vi "IEEE754-V1.1.vi"(3 "error in (no error)":errorcluster caption="错误输入（无错误）", 5 "数字":i32 format="%.0x") -> (0 "error out":errorcluster caption="错误输出", 2 "输出浮点型":dbl)   [LabVIEW 2015]
panel:
  out "HexFormat":i32=1130102784 format="%x"
  # "IEEE754 2个16位整型转换为浮点型"
  # "1、程序将两个16位整型转换为一个32为的浮点型数据，转换原则按照IEEE754标准进行；\n2、高16、低16位和合并后的Hex格式数据都是16进制显示；\n3、输出浮点型是转换后的数据。"
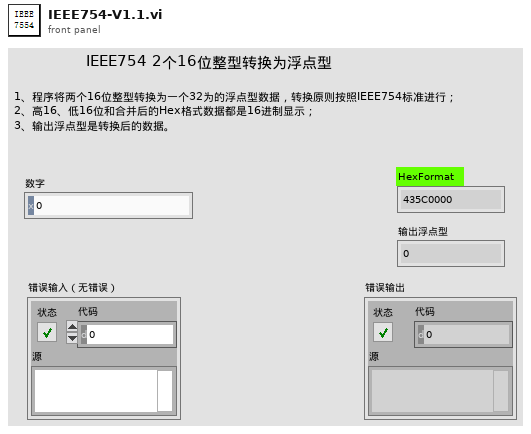
[diagram p1: front panel]
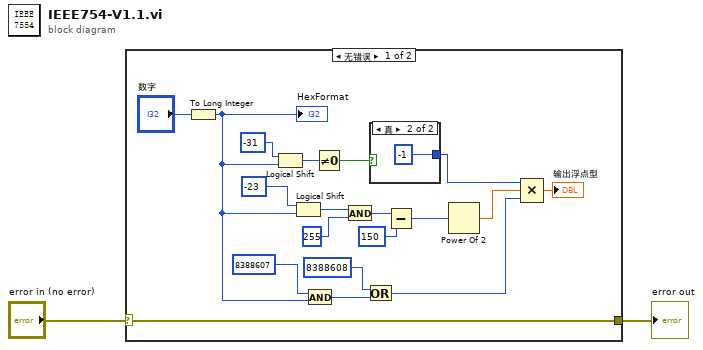
[diagram p0: block diagram]
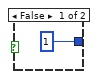
[diagram p2: hidden frame]
diagram:
  n1 = case shown="无错误" "error in (no error)" {
    selector: "error in (no error)" -> [w3 w24]
    tunnel: [w3 w24] -> w1
    frame No Error {
      n2 = To Long Integer(number="数字") -> (32bit integer=w5:i32)
      "HexFormat" <- w5
      n3 = Logical Shift(y=-31, x=w5) -> (x << y=w20:i32)
      n4 = Logical Shift(y=-23, x=w5) -> (x << y=w17:i32)
      n5 = And(x=8388607, y=w5) -> (x .and. y?=w12:i32)
      n6 = Not Equal To 0?(x=w20) -> (x != 0?=w19:bool)
      n7 = And(x=w17, y=255) -> (x .and. y?=w15:i32)
      n8 = Or(x=8388608, y=w12) -> (x .or. y?=w9:i32)
      n9 = case shown="真" w19 {
        tunnel: [1 -1] -> w10
        frame False {
        }
        frame True {
        }
      }
      n10 = Subtract(x=w15, y=150) -> (x-y=w7:i32)
      n11 = Power Of 2(x=w7) -> (2^x=w6:dbl)
      n12 = Compound Arithmetic op=MULTIPLY(w10, w6, w9) -> (→"输出浮点型":dbl)
    }
    frame Error {
    }
  }
  "error out" <- w1
